vi "Read N Screen Taps.vi"(8 "Error In":errorcluster, 11 "Leap Handle":T6) -> (0 "Error Out":errorcluster, 1 "Screen Tap Statuses":T1[](array[typedef]), 2 "Screen Tap Gestures":T2[](array[typedef]), 3 "Leap Handle":T6)   [LabVIEW 2014, in "LMH-Leap.lvlib"]
doc: "Read all data from N screen tap gestures."
uses:
  LMH-Leap.lvlib
  Private/Type Defs/Leap Handle.ctl
  C:/github/makerhub/Leap/LabVIEW/vi.lib/LabVIEW Hacker/Leap/Private/Libs/LeapCSharp.NET3.5.dll
  LabVIEW Hacker/Leap/Private/Libs/LeapCSharp.NET3.5.dll
  Private/Type Defs/Gesture Screen Tap.ctl
  Private/Type Defs/Gesture Common.ctl
  Private/Type Defs/Gesture Type.ctl
  Private/Type Defs/Gesture State.ctl
  Private/Type Defs/Vector.ctl
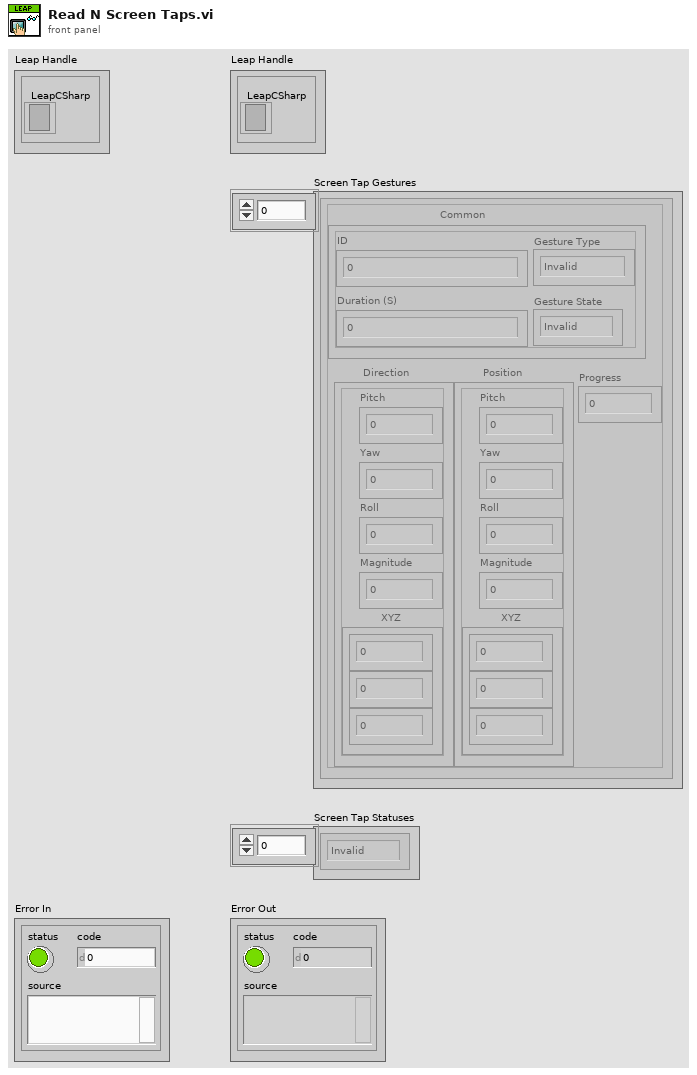
[diagram p1: front panel]
types:
  T1 = typedef "LMH-Leap.lvlib/Gesture State.ctl" = enum16{"Invalid", "Start", "Update", "Stop"}
  T2 = typedef "LMH-Leap.lvlib/Gesture Screen Tap.ctl" = cluster{"Common":T3, "Direction":T5, "Position":T5, "Progress":dbl}
  T3 = typedef "LMH-Leap.lvlib/Gesture Common.ctl" = cluster{"ID":dbl, "Duration (S)":dbl, "Gesture Type":T4, "Gesture State":T1}
  T4 = typedef "LMH-Leap.lvlib/Gesture Type.ctl" = enum16{"Invalid", "Swipe", "Circle", "Screen Tap", "Key Tap"}
  T5 = typedef "LMH-Leap.lvlib/Vector.ctl" = cluster{"Pitch":sgl, "Yaw":sgl, "Roll":sgl, "Magnitude":sgl, "XYZ":sgl[]}
  T6 = typedef "LMH-Leap.lvlib/Leap Handle.ctl" = cluster{"LeapCSharp":refnum<k24>}
  T7 = typedef "LMH-Leap.lvlib/Frame.ctl" = cluster{"ID":i64, "Timestamp":i64, "Current FPS":dbl, "Key Tap Gestures":T8[], "Circle Gestures":T9[], "Screen Tap Gestures":T2[], "Swipe Gestures":T10[], "Hands":T11[]}
  T8 = typedef "LMH-Leap.lvlib/Gesture Key Tap.ctl" = cluster{"Common":T3, "Direction":T5, "Position":T5, "Progress":dbl}
  T9 = typedef "LMH-Leap.lvlib/Gesture Circle.ctl" = cluster{"Common":T3, "Center":T5, "Normal":T5, "Progress":dbl, "Radius":dbl}
  T10 = typedef "LMH-Leap.lvlib/Gesture Swipe.ctl" = cluster{"Common":T3, "Direction":T5, "Position":T5, "Start Position":T5, "Speed":dbl}
  T11 = typedef "LMH-Leap.lvlib/Hand.ctl" = cluster{"Palm Normal":T5, "Palm Position":T5, "Palm Velocity":T5, "Direction":T5, "Palm Position (Stabilized)":T5, "Sphere Center":T5, "Pointables":T12[], "ID":i32, "Time Visible":sgl, "Sphere Radius":sgl}
  T12 = typedef "LMH-Leap.lvlib/Pointable.ctl" = cluster{"Type":T13, "Touch Zone":T14, "ID":i32, "Length":dbl, "Width":dbl, "Time Visible":dbl, "Touch Distance":dbl, "Direction":T5, "Tip Position":T5, "Tip Velocity":T5, "Tip Position (Stabilized)":T5}
  T13 = typedef "LMH-Leap.lvlib/Pointable Type.ctl" = enum16{"Finger", "Tool"}
  T14 = typedef "LMH-Leap.lvlib/Pointable Zone.ctl" = enum16{"None", "Hovering", "Touching"}
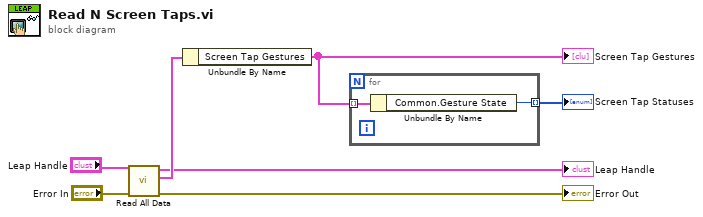
[diagram p0: block diagram]
diagram:
  n1 = call "Read All Data.vi"("Error In"="Error In", "Leap Handle"="Leap Handle") -> ("Error Out"=→"Error Out":errorcluster, "Frame"=w7:T7, "Leap Handle"=→"Leap Handle":T6)  [unwired: 6 in, 1 out]
  n2 = Unbundle By Name(w7) -> ("Screen Tap Gestures"=w1:T2[])
  "Screen Tap Gestures" <- w1
  n3 = for {
    tunnel: w1 -> [w9] mode=indexing
    tunnel: [w8] -> w2 mode=indexing
    n4 = Unbundle By Name(w9) -> ("Common.Gesture State"=w8:T1)
  }
  "Screen Tap Statuses" <- w2
